vi "New.vi"(3 "Colour":u32(colorbox), 5 "error in (no error)":errorcluster) -> (14 "object out":refnum<class "Fruit.lvclass">, 19 "error out":errorcluster)   [LabVIEW 2021, in "Fruit.lvclass"]
uses:
  Fruit.lvclass
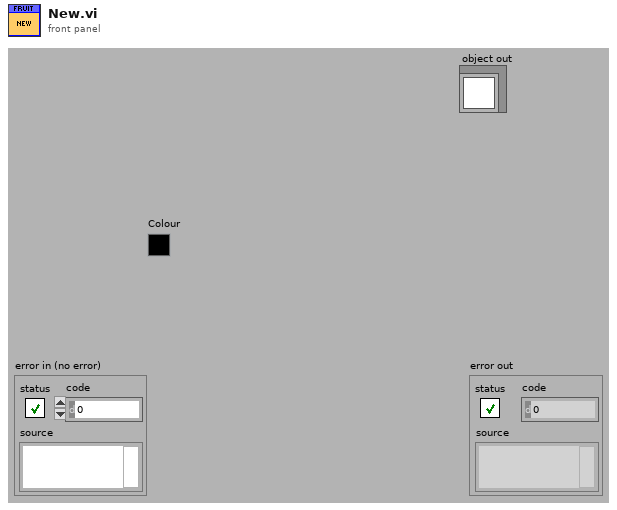
[diagram p1: front panel]
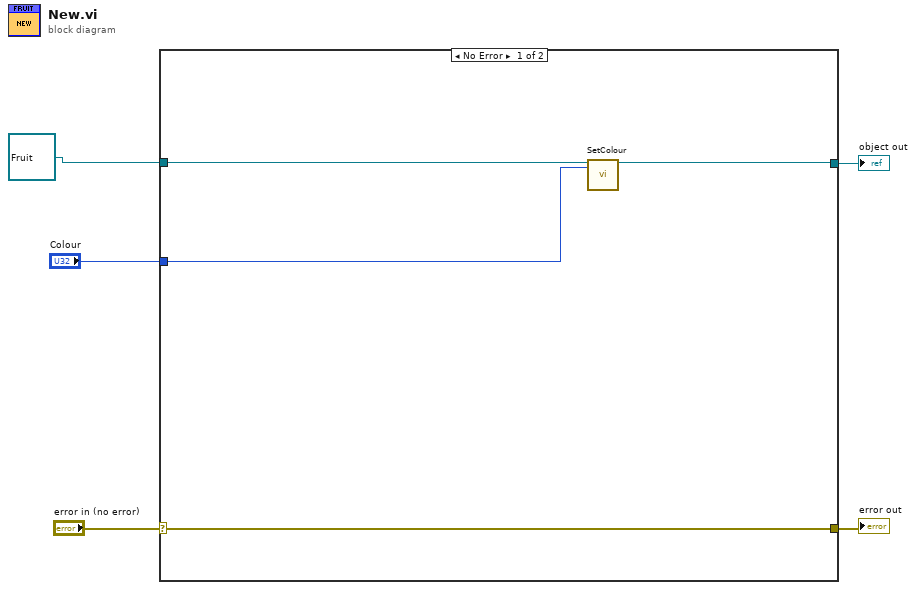
[diagram p0: block diagram]
diagram:
  n1 = case shown="No Error" "error in (no error)" {
    selector: "error in (no error)" -> [w9 w11]
    tunnel: [w9 w11] -> w4
    tunnel: [w6 w10] -> w3
    tunnel: refnum<class "Fruit.lvclass"> refnum ("Fruit") -> [w8 w10]
    tunnel: "Colour" -> [w7 _]
    frame No Error {
      n2 = call-dynamic "SetColour.vi"("object in"=w8, "Colour"=w7) -> ("object out"=w6:refnum<class "Fruit.lvclass">)  [unwired: 16 in, 1 out]
    }
    frame Error {
    }
  }
  "error out" <- w4
  "object out" <- w3
